vi "TCPtaskhandle.vi"(6 "心跳包":refnum<vi>, 9 "配置信息":refnum<vi>, 10 "状态信息":refnum<vi>, 11 "通信状态":refnum<vi>) -> ()   [LabVIEW 2016, in "数据传输系统.lvlib"]
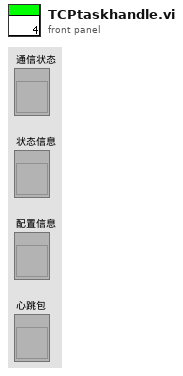
[diagram p1: front panel]
types:
  T1 = cluster{"setini":string, "sysini":string, "hechaini":string, "actualwrite":string, "actualread":string, "datasent":string, "反控命令信息队列":string, "反控与仪器交互":string}
  T2 = cluster{"站点":string, "设备":string, "IP":string, "PORT":string, "MN":string, "PW":string}
  T3 = cluster{"1st Error to Convert ":i32, "步骤 ":enum16{"打开连接", "发送数据", "读取数据", "数据处理", "关闭连接"}, "元素":string, "TCP服务端掉线计数":i32, "TCP掉线时间节点":string}
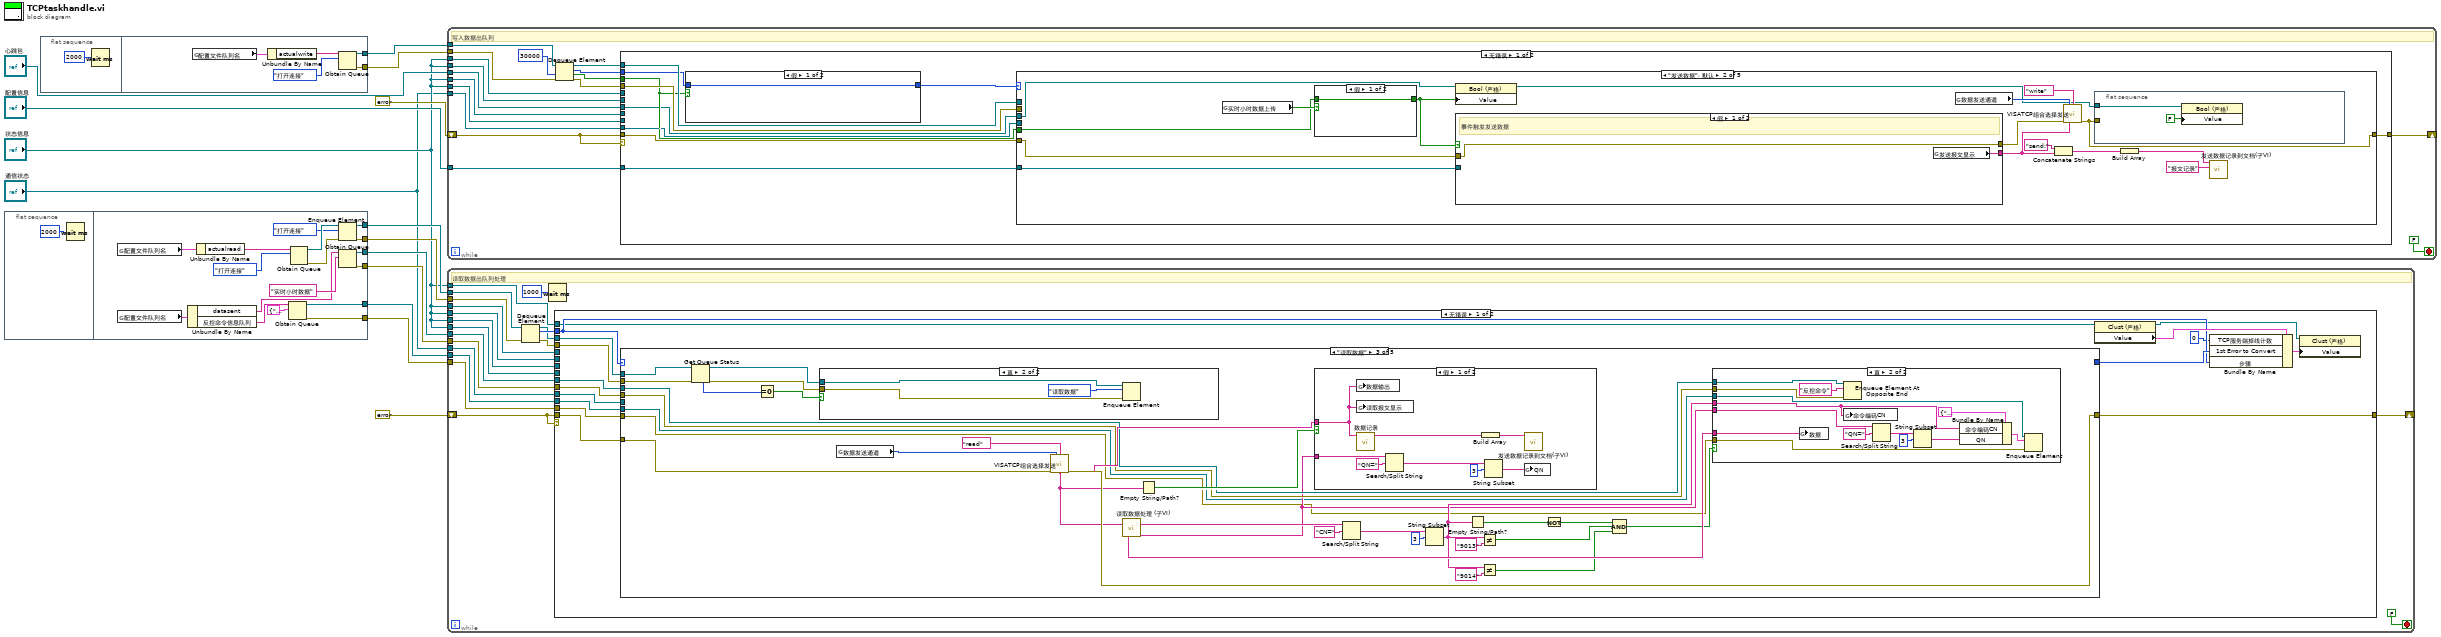
[diagram p0: block diagram]
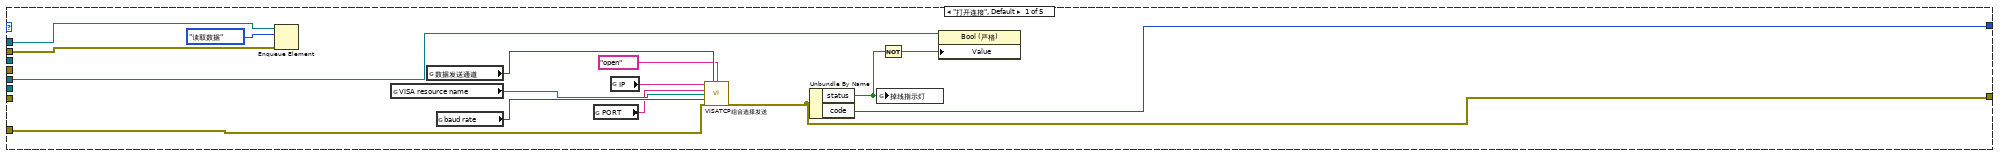
[diagram p2: hidden frame]
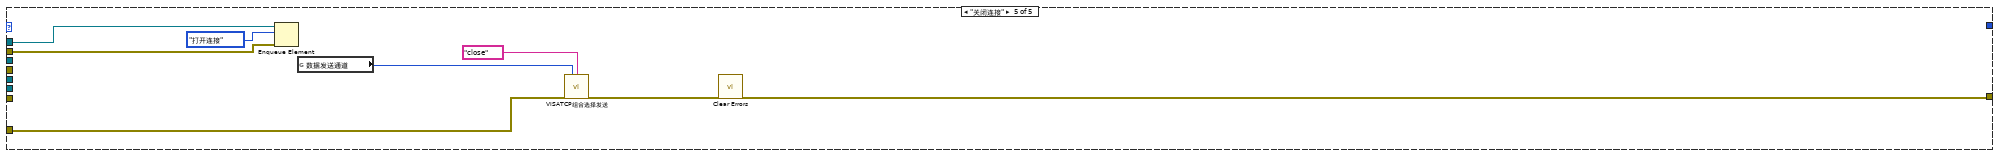
[diagram p8: hidden frame]
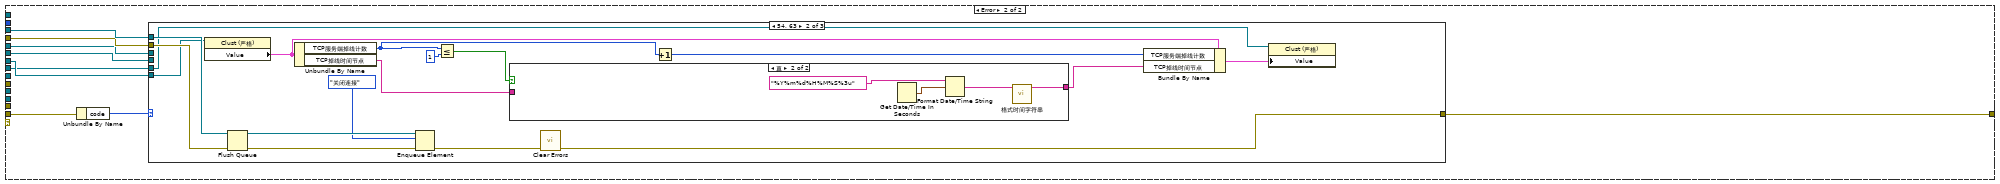
[diagram p9: hidden frame]
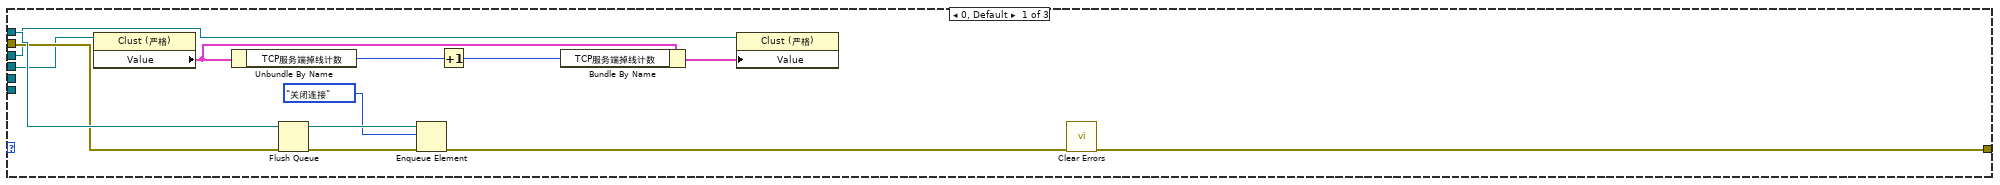
[diagram p10: hidden frame]
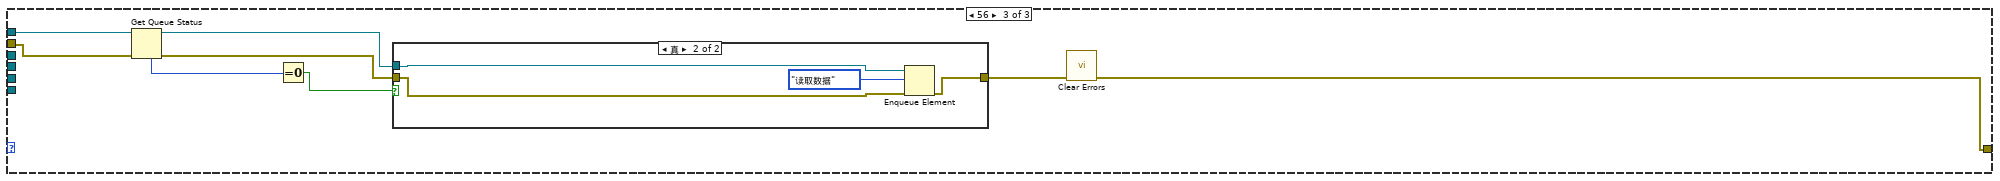
[diagram p12: hidden frame]
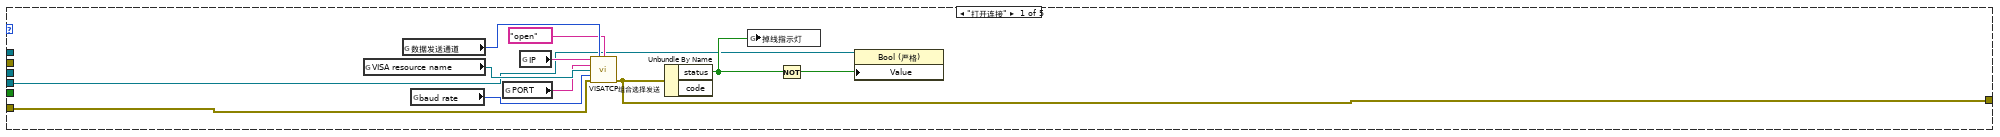
[diagram p14: hidden frame]
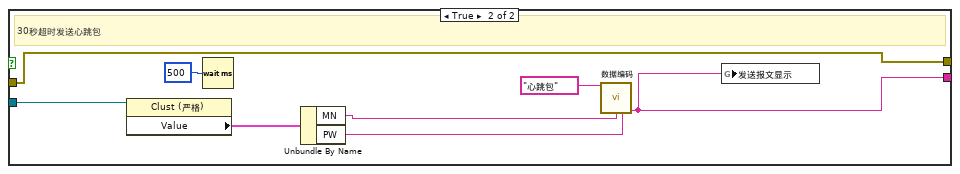
[diagram p15: hidden frame]
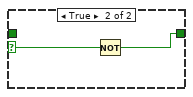
[diagram p16: hidden frame]
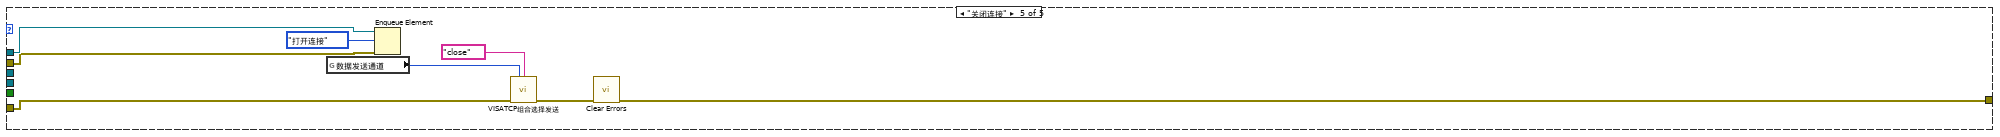
[diagram p19: hidden frame]
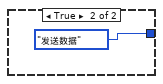
[diagram p20: hidden frame]
diagram:
  n1 = flat-sequence {
    tunnel: [w29] -> w8
    tunnel: [w28] -> w9
    tunnel: [w26] -> w11
    tunnel: [w25] -> w12
    tunnel: [w23] -> w13
    tunnel: [w22] -> w14
    frame #0 {
      n2 = Wait (ms)(milliseconds to wait=u32 2000 ("等待时间（毫秒）")) -> ()  [unwired: 1 out]
    }
    frame #1 {
      n3 = global read "断电保存全局.vi" "配置文件队列名"() -> (w20:T1)
      n4 = global read "断电保存全局.vi" "配置文件队列名"() -> (w18:T1)
      n5 = Unbundle By Name(w18) -> ("datasent"=w17:string, "反控命令信息队列"=w16:string)
      n6 = Unbundle By Name(w20) -> ("actualread"=w19:string)
      n7 = Obtain Queue(name (unnamed)=w16, element data type=cluster{"命令编码CN":string, "QN":string} {"命令编码CN"="", "QN"=""}) -> (queue out=w23:refnum<queue>, error out=w22:errorcluster)  [unwired: 3 in, 1 out]
      n8 = Obtain Queue(name (unnamed)=w19, element data type=enum16{"打开连接", "发送数据", "读取数据", "数据处理", "关闭连接"}."打开连接" ("枚举")) -> (queue out=w32:refnum<queue>, error out=w27:errorcluster)  [unwired: 3 in, 1 out]
      n9 = Enqueue Element(queue=w32, element=enum16{"打开连接", "发送数据", "读取数据", "数据处理", "关闭连接"}."打开连接" ("枚举"), error in (no error)=w27) -> (queue out=w29:refnum<queue>, error out=w28:errorcluster)  [unwired: 1 in, 1 out]
      n10 = Obtain Queue(name (unnamed)=w17, element data type="实时小时数据" ("元素")) -> (queue out=w26:refnum<queue>, error out=w25:errorcluster)  [unwired: 3 in, 1 out]
    }
  }
  n11 = flat-sequence {
    tunnel: [w37] -> w5
    tunnel: [w36] -> w6
    frame #0 {
      n12 = Wait (ms)(milliseconds to wait=u32 2000 ("等待时间（毫秒）")) -> ()  [unwired: 1 out]
    }
    frame #1 {
      n13 = global read "断电保存全局.vi" "配置文件队列名"() -> (w35:T1)
      n14 = Unbundle By Name(w35) -> ("actualwrite"=w34:string)
      n15 = Obtain Queue(name (unnamed)=w34, element data type=enum16{"打开连接", "发送数据", "读取数据", "数据处理", "关闭连接"}."打开连接" ("枚举")) -> (queue out=w37:refnum<queue>, error out=w36:errorcluster)  [unwired: 3 in, 1 out]
    }
  }
  n16 = while {
    tunnel: w5 -> [w54]
    tunnel: w6 -> [w53]
    shift-right: [w49] -> _
    shift-left: errorcluster {"status"=FALSE, "code"=0, "source"=""} ("error out") -> [w48]
    tunnel: "通信状态" -> [w45]
    tunnel: "配置信息" -> [w44]
    tunnel: "心跳包" -> [w43]
    tunnel: "状态信息" -> [w42]
    tunnel: "状态信息" -> [w41]
    tunnel: "状态信息" -> [w40]
    tunnel: "状态信息" -> [w39]
    stop <- FALSE stop-if-true
    # "写入数据出队列"
    n17 = Dequeue Element(queue=w54, timeout in ms (-1)=30000 ("超时毫秒(-1)"), error in (no error)=w53) -> (queue out=w47:refnum<queue>, element=w51:enum16{"打开连接", "发送数据", "读取数据", "数据处理", "关闭连接"}, timed out?=w50:bool, error out=w46:errorcluster)
    n18 = case shown="无错误" w48 {
      tunnel: w51 -> [w59 _]
      tunnel: w50 -> [w61 _]
      tunnel: [w65 w122] -> w49
      tunnel: w48 -> [w64 w126]
      tunnel: w47 -> [w63 w124]
      tunnel: w46 -> [w62 w123]
      tunnel: w45 -> [w58 _]
      tunnel: w44 -> [w57 _]
      tunnel: w43 -> [w56 _]
      tunnel: w42 -> [_ w121]
      tunnel: w41 -> [_ w120]
      tunnel: w40 -> [_ w119]
      tunnel: w39 -> [_ w118]
      frame No Error {
        n19 = case shown="假" w61 {
          tunnel: [w116 enum16{"打开连接", "发送数据", "读取数据", "数据处理", "关闭连接"}."发送数据" ("枚举")] -> w60
          tunnel: w59 -> [w116 _]
          frame False {
          }
          frame True {
          }
        }
        n20 = case shown="\"发送数据\", 默认" w60 {
          tunnel: w61 -> [_ w81 _ _ _]
          tunnel: [w68 w84 _ _ w109] -> w65
          tunnel: w64 -> [w70 w90 _ _ w110]
          tunnel: w63 -> [_ _ _ _ w111]
          tunnel: w62 -> [_ _ _ _ w108]
          tunnel: w58 -> [w66 _ _ _ _]
          tunnel: w57 -> [_ w80 _ _ _]
          tunnel: w56 -> [_ w78 _ _ _]
          frame "打开连接" {
            n21 = global read "断电保存全局.vi" "VISA resource name"() -> (w76:refnum<visa-resource-name>)
            n22 = global read "断电保存全局.vi" "数据发送通道"() -> (w73:enum16{"TCP", "VISA"})
            n23 = global read "断电保存全局.vi" "baud rate"() -> (w75:u32)
            n24 = global read "断电保存全局.vi" "PORT"() -> (w74:string)
            n25 = global read "断电保存全局.vi" "IP"() -> (w72:string)
            n26 = call "VISATCP组合选择发送.vi"("IP"=w72, "数据发送通道"=w73, "命令"="open", "PORT"=w74, "VISA resource name"=w76, "baud rate"=w75, "error in (no error)"=w70) -> ("错误输出"=w68:errorcluster)  [unwired: 5 in, 3 out]
            n27 = Unbundle By Name(w68) -> ("status"=w67:bool)  [unwired: 1 out]
            n28 = global write "全局 数据发送重叠.vi" "掉线指示灯"(w67) -> ()
            n29 = Not(x=w67) -> (.not. x?=w69:bool)
            n30 = property class="Bool (严格)"(reference=w66, "Value"=w69) -> ()  [unwired: 1 in, 2 out]
          }
          frame "发送数据", Default {
            n31 = global read "全局1.vi" "实时小时数据上传"() -> (w82:bool)
            n32 = case shown="假" w82 {
              selector: w82 -> [_ w107]
              tunnel: w81 -> [w105 _]
              tunnel: [w105 w106] -> w79
              frame False {
              }
              frame True {
                n33 = Not(x=w107) -> (.not. x?=w106:bool)
              }
            }
            n34 = property class="Bool (严格)"(reference=w78, "Value"=w79) -> (reference out=w77:refnum<vi>)  [unwired: 1 in, 1 out]
            n35 = case shown="假" w79 {
              tunnel: [w96 w99] -> w86
              tunnel: w90 -> [w95 w100]
              tunnel: [w95 w100] -> w89
              tunnel: w80 -> [_ w97]
              frame False {
                # "事件触发发送数据"
                n36 = global read "全局1.vi" "发送报文显示"() -> (w96:string)
              }
              frame True {
                # "30秒超时发送心跳包"
                n37 = property class="Clust (严格)"(reference=w97) -> ("Value"=w103:T2)  [unwired: 1 in, 2 out]
                n38 = Wait (ms)(milliseconds to wait=u32 500 ("等待时间（毫秒）")) -> ()  [unwired: 1 out]
                n39 = Unbundle By Name(w103) -> ("MN"=w102:string, "PW"=w101:string)
                n40 = call "数据编码.vi"("table输入"="心跳包", "MN"=w102, "PW"=w101) -> ("通讯包字符串"=w99:string)  [unwired: 11 in, 1 out]
                n41 = global write "全局1.vi" "发送报文显示"(w99) -> ()
              }
            }
            n42 = global read "断电保存全局.vi" "数据发送通道"() -> (w91:enum16{"TCP", "VISA"})
            n43 = Concatenate Strings("send:" ("字符串"), w86) -> (w85:string)
            n44 = call "VISATCP组合选择发送.vi"("数据发送通道"=w91, "命令"="write", "error in (no error)"=w89, "写入缓冲区"=w86) -> ("错误输出"=w84:errorcluster)  [unwired: 8 in, 3 out]
            n45 = flat-sequence {
              tunnel: w84 -> [_]
              tunnel: w77 -> [w93]
              frame #0 {
                n46 = property class="Bool (严格)"(reference=w93, "Value"=FALSE ("心跳包")) -> ()  [unwired: 1 in, 2 out]
              }
            }
            n47 = Build Array(w85) -> (w88:string[])
            n48 = call "发送数据记录到文档(子VI).vi"("字符串"="报文记录", "数组"=w88) -> ()  [unwired: 8 in, 1 out]
          }
          frame "读取数据" {
          }
          frame "数据处理" {
          }
          frame "关闭连接" {
            n49 = global read "断电保存全局.vi" "数据发送通道"() -> (w113:enum16{"TCP", "VISA"})
            n50 = Enqueue Element(queue=w111, element=enum16{"打开连接", "发送数据", "读取数据", "数据处理", "关闭连接"}."打开连接" ("枚举"), error in (no error)=w108) -> ()  [unwired: 1 in, 3 out]
            n51 = call "VISATCP组合选择发送.vi"("数据发送通道"=w113, "命令"="close", "error in (no error)"=w110) -> ("错误输出"=w114:errorcluster)  [unwired: 9 in, 3 out]
            n52 = call <vilib>:"Clear Errors.vi"("error in (no error)"=w114) -> ("error out"=w109:errorcluster)  [unwired: 5 in, 1 out]
          }
        }
      }
      frame Error {
        n53 = Unbundle By Name(w126) -> ("code"=w125:i32)
        n54 = case shown="54, 63" w125 {
          tunnel: w124 -> [w135 w153 w165]
          tunnel: w123 -> [w134 w152 w164]
          tunnel: [w133 w150 w163] -> w122
          tunnel: w121 -> [w128 _ _]
          tunnel: w120 -> [w127 _ _]
          tunnel: w119 -> [_ w141 _]
          tunnel: w118 -> [_ w140 _]
          frame 0, Default {
            n55 = property class="Clust (严格)"(reference=w128) -> ("Value"=w132:T3)  [unwired: 1 in, 2 out]
            n56 = Unbundle By Name(w132) -> ("TCP服务端掉线计数"=w130:i32)
            n57 = Flush Queue(queue=w135, error in (no error)=w134) -> (queue out=w137:refnum<queue>, error out=w138:errorcluster)  [unwired: 1 out]
            n58 = Enqueue Element(queue=w137, element=enum16{"打开连接", "发送数据", "读取数据", "数据处理", "关闭连接"}."关闭连接" ("枚举"), error in (no error)=w138) -> (error out=w139:errorcluster)  [unwired: 1 in, 2 out]
            n59 = Increment(x=w130) -> (x+1=w131:i32)
            n60 = Bundle By Name(cluster=w132, "TCP服务端掉线计数"=w131) -> (w129:T3)
            n61 = property class="Clust (严格)"(reference=w127, "Value"=w129) -> ()  [unwired: 1 in, 2 out]
            n62 = call <vilib>:"Clear Errors.vi"("error in (no error)"=w139) -> ("error out"=w133:errorcluster)  [unwired: 5 in, 1 out]
          }
          frame 54, 63 {
            n63 = property class="Clust (严格)"(reference=w141) -> ("Value"=w145:T3)  [unwired: 1 in, 2 out]
            n64 = Flush Queue(queue=w153, error in (no error)=w152) -> (queue out=w155:refnum<queue>, error out=w156:errorcluster)  [unwired: 1 out]
            n65 = Unbundle By Name(w145) -> ("TCP服务端掉线计数"=w149:i32, "TCP掉线时间节点"=w142:string)
            n66 = Enqueue Element(queue=w155, element=enum16{"打开连接", "发送数据", "读取数据", "数据处理", "关闭连接"}."关闭连接" ("枚举"), error in (no error)=w156) -> (error out=w151:errorcluster)  [unwired: 1 in, 2 out]
            n67 = Less Or Equal?(x=w149, y=1) -> (x <= y?=w147:bool)
            n68 = case shown="真" w147 {
              tunnel: [w157 w158] -> w146
              tunnel: w142 -> [w157 _]
              frame False {
              }
              frame True {
                n69 = Get Date/Time In Seconds() -> (seconds since 1Jan1904=w159:timestamp)
                n70 = Format Date/Time String(time format string (%c)="%Y%m%d%H%M%S%3u" ("时间格式字符串(%c)"), seconds (now)=w159) -> (date/time string=w161:string)  [unwired: 1 in]
                n71 = call "格式时间字符串.vi"("字符串"=w161) -> ("连接的字符串"=w158:string)  [unwired: 10 in]
              }
            }
            n72 = call <vilib>:"Clear Errors.vi"("error in (no error)"=w151) -> ("error out"=w150:errorcluster)  [unwired: 5 in, 1 out]
            n73 = Increment(x=w149) -> (x+1=w144:i32)
            n74 = Bundle By Name(cluster=w145, "TCP服务端掉线计数"=w144, "TCP掉线时间节点"=w146) -> (w143:T3)
            n75 = property class="Clust (严格)"(reference=w140, "Value"=w143) -> ()  [unwired: 1 in, 2 out]
          }
          frame 56 {
            n76 = Flush Queue(queue=w165, error in (no error)=w164) -> (error out=w162:errorcluster)  [unwired: 2 out]
            n77 = call <vilib>:"Clear Errors.vi"("error in (no error)"=w162) -> ("error out"=w163:errorcluster)  [unwired: 5 in, 1 out]
          }
        }
      }
    }
  }
  n78 = while {
    tunnel: w8 -> [w184]
    tunnel: w9 -> [w183]
    shift-right: [w180] -> _
    shift-left: errorcluster {"status"=FALSE, "code"=0, "source"=""} ("error out") -> [w179]
    tunnel: w11 -> [w175]
    tunnel: w12 -> [w174]
    tunnel: w13 -> [w173]
    tunnel: w14 -> [w172]
    tunnel: "状态信息" -> [w171]
    tunnel: "状态信息" -> [w170]
    tunnel: "状态信息" -> [w169]
    tunnel: "状态信息" -> [w168]
    tunnel: "状态信息" -> [w167]
    tunnel: "通信状态" -> [w166]
    stop <- FALSE stop-if-true
    # "读取数据出队列处理"
    n79 = Dequeue Element(queue=w184, error in (no error)=w183) -> (queue out=w178:refnum<queue>, element=w181:enum16{"打开连接", "发送数据", "读取数据", "数据处理", "关闭连接"}, error out=w177:errorcluster)  [unwired: 1 in, 1 out]
    n80 = Wait (ms)(milliseconds to wait=u32 1000 ("等待时间（毫秒）")) -> ()  [unwired: 1 out]
    n81 = case shown="无错误" w179 {
      tunnel: w181 -> [w194 _]
      tunnel: [w200 w283] -> w180
      tunnel: w179 -> [w199 w287]
      tunnel: w178 -> [w198 w285]
      tunnel: w177 -> [w197 w284]
      tunnel: w175 -> [w192 _]
      tunnel: w174 -> [w191 _]
      tunnel: w173 -> [w190 _]
      tunnel: w172 -> [w189 _]
      tunnel: w171 -> [w188 _]
      tunnel: w170 -> [_ w282]
      tunnel: w169 -> [_ w281]
      tunnel: w168 -> [_ w280]
      tunnel: w167 -> [_ w279]
      tunnel: w166 -> [w185 _]
      frame No Error {
        n82 = case shown="\"读取数据\"" w194 {
          tunnel: [w209 _ w242 _ w274] -> w200
          tunnel: w199 -> [w208 _ w245 _ w275]
          tunnel: w198 -> [w206 _ w237 _ w272]
          tunnel: w197 -> [w205 _ w236 _ w271]
          tunnel: [w204 _ _ _ _] -> w195
          tunnel: w192 -> [_ _ w229 _ _]
          tunnel: w191 -> [_ _ w228 _ _]
          tunnel: w190 -> [_ _ w217 _ _]
          tunnel: w189 -> [_ _ w216 _ _]
          tunnel: w185 -> [w202 _ _ _ _]
          frame "打开连接", Default {
            n83 = Enqueue Element(queue=w206, element=enum16{"打开连接", "发送数据", "读取数据", "数据处理", "关闭连接"}."读取数据" ("枚举"), error in (no error)=w205) -> ()  [unwired: 1 in, 3 out]
            n84 = global read "断电保存全局.vi" "VISA resource name"() -> (w215:refnum<visa-resource-name>)
            n85 = global read "断电保存全局.vi" "数据发送通道"() -> (w212:enum16{"TCP", "VISA"})
            n86 = global read "断电保存全局.vi" "baud rate"() -> (w214:u32)
            n87 = global read "断电保存全局.vi" "PORT"() -> (w213:string)
            n88 = global read "断电保存全局.vi" "IP"() -> (w211:string)
            n89 = call "VISATCP组合选择发送.vi"("IP"=w211, "数据发送通道"=w212, "命令"="open", "PORT"=w213, "VISA resource name"=w215, "baud rate"=w214, "error in (no error)"=w208) -> ("错误输出"=w209:errorcluster)  [unwired: 5 in, 3 out]
            n90 = Unbundle By Name(w209) -> ("status"=w203:bool, "code"=w204:i32)
            n91 = global write "全局 数据发送重叠.vi" "掉线指示灯"(w203) -> ()
            n92 = Not(x=w203) -> (.not. x?=w201:bool)
            n93 = property class="Bool (严格)"(reference=w202, "Value"=w201) -> ()  [unwired: 1 in, 2 out]
          }
          frame "发送数据" {
          }
          frame "读取数据" {
            n94 = Get Queue Status(queue=w237, error in (no error)=w236) -> (queue out=w233:refnum<queue>, error out=w232:errorcluster, # elements in queue=w235:i32)  [unwired: 1 in, 5 out]
            n95 = Equal To 0?(x=w235) -> (x = 0?=w234:bool)
            n96 = case shown="真" w234 {
              tunnel: w233 -> [_ w269]
              tunnel: w232 -> [_ w268]
              frame False {
              }
              frame True {
                n97 = Enqueue Element(queue=w269, element=enum16{"打开连接", "发送数据", "读取数据", "数据处理", "关闭连接"}."读取数据" ("枚举"), error in (no error)=w268) -> ()  [unwired: 1 in, 3 out]
              }
            }
            n98 = global read "断电保存全局.vi" "数据发送通道"() -> (w244:enum16{"TCP", "VISA"})
            n99 = call "VISATCP组合选择发送.vi"("数据发送通道"=w244, "命令"="read", "error in (no error)"=w245) -> ("读取缓冲区"=w230:string, "错误输出"=w242:errorcluster)  [unwired: 9 in, 2 out]
            n100 = call "读取数据处理 (子VI).vi"("data out"=w230) -> ("命令编码CN"=w238:string, "数据"=w226:string, "时间QN"=w218:string)  [unwired: 8 in, 4 out]
            n101 = Empty String/Path?(string/path=w230) -> (empty?=w231:bool)
            n102 = case shown="假" w231 {
              tunnel: w230 -> [w265 _]
              tunnel: w218 -> [w262 _]
              frame False {
                n103 = global write "全局1.vi" "数据输出"(w265) -> ()
                n104 = global write "全局1.vi" "读取报文显示"(w265) -> ()
                n105 = call "数据记录.vi"("写入字段"=w265) -> ("连接的字符串"=w266:string)  [unwired: 10 in]
                n106 = Search/Split String(string=w262, search string/char (-)="QN=" ("搜索字符串/字符(-)")) -> (match + rest of string=w261:string)  [unwired: 1 in, 2 out]
                n107 = Build Array(w266) -> (w267:string[])
                n108 = String Subset(string=w261, offset (0)=3 ("偏移量(0)")) -> (substring=w260:string)  [unwired: 1 in]
                n109 = call "发送数据记录到文档(子VI).vi"("数组"=w267) -> ()  [unwired: 9 in, 1 out]
                n110 = global write "全局1.vi" "QN"(w260) -> ()
              }
              frame True {
              }
            }
            n111 = Search/Split String(string=w238, search string/char (-)="CN=" ("搜索字符串/字符(-)")) -> (match + rest of string=w239:string)  [unwired: 1 in, 2 out]
            n112 = String Subset(string=w239, offset (0)=3 ("偏移量(0)")) -> (substring=w224:string)  [unwired: 1 in]
            n113 = Empty String/Path?(string/path=w224) -> (empty?=w227:bool)
            n114 = Not Equal?(x=w224, y="9013") -> (x != y?=w221:bool)
            n115 = Not Equal?(x=w224, y="9014") -> (x != y?=w220:bool)
            n116 = Not(x=w227) -> (.not. x?=w219:bool)
            n117 = Compound Arithmetic op=AND ("复合运算")(w219, w221, w220) -> (w225:bool)
            n118 = case shown="真" w225 {
              tunnel: w229 -> [_ w259]
              tunnel: w228 -> [_ w258]
              tunnel: w226 -> [_ w257]
              tunnel: w224 -> [_ w248]
              tunnel: w218 -> [_ w253]
              tunnel: w217 -> [_ w252]
              tunnel: w216 -> [_ w251]
              frame False {
              }
              frame True {
                n119 = global write "全局1.vi" "数据"(w257) -> ()
                n120 = Enqueue Element At Opposite End(queue=w259, element="反控命令" ("元素"), error in (no error)=w258) -> ()  [unwired: 1 in, 3 out]
                n121 = global write "全局1.vi" "命令编码CN"(w248) -> ()
                n122 = Search/Split String(string=w253, search string/char (-)="QN=" ("搜索字符串/字符(-)")) -> (match + rest of string=w256:string)  [unwired: 1 in, 2 out]
                n123 = String Subset(string=w256, offset (0)=3 ("偏移量(0)")) -> (substring=w247:string)  [unwired: 1 in]
                n124 = Bundle By Name(cluster=cluster{"命令编码CN":string, "QN":string} {"命令编码CN"="", "QN"=""}, "命令编码CN"=w248, "QN"=w247) -> (w249:cluster{"命令编码CN":string, "QN":string})
                n125 = Enqueue Element(queue=w252, element=w249, error in (no error)=w251) -> ()  [unwired: 1 in, 3 out]
              }
            }
          }
          frame "数据处理" {
          }
          frame "关闭连接" {
            n126 = Enqueue Element(queue=w272, element=enum16{"打开连接", "发送数据", "读取数据", "数据处理", "关闭连接"}."打开连接" ("枚举"), error in (no error)=w271) -> ()  [unwired: 1 in, 3 out]
            n127 = global read "断电保存全局.vi" "数据发送通道"() -> (w277:enum16{"TCP", "VISA"})
            n128 = call "VISATCP组合选择发送.vi"("数据发送通道"=w277, "命令"="close", "error in (no error)"=w275) -> ("错误输出"=w276:errorcluster)  [unwired: 9 in, 3 out]
            n129 = call <vilib>:"Clear Errors.vi"("error in (no error)"=w276) -> ("error out"=w274:errorcluster)  [unwired: 5 in, 1 out]
          }
        }
        n130 = property class="Clust (严格)"(reference=w188) -> (reference out=w187:refnum<vi>, "Value"=w196:T3)  [unwired: 1 in, 1 out]
        n131 = Bundle By Name(cluster=w196, "TCP服务端掉线计数"=0, "1st Error to Convert"=w195, "步骤"=w194) -> (w186:T3)
        n132 = property class="Clust (严格)"(reference=w187, "Value"=w186) -> ()  [unwired: 1 in, 2 out]
      }
      frame Error {
        n133 = Unbundle By Name(w287) -> ("code"=w286:i32)
        n134 = case shown="54, 63" w286 {
          tunnel: w285 -> [w296 w314 w324]
          tunnel: w284 -> [w295 w313 w323]
          tunnel: [w294 w311 w330] -> w283
          tunnel: w282 -> [w289 _ _]
          tunnel: w281 -> [w288 _ _]
          tunnel: w280 -> [_ w302 _]
          tunnel: w279 -> [_ w301 _]
          frame 0, Default {
            n135 = property class="Clust (严格)"(reference=w289) -> ("Value"=w293:T3)  [unwired: 1 in, 2 out]
            n136 = Unbundle By Name(w293) -> ("TCP服务端掉线计数"=w291:i32)
            n137 = Flush Queue(queue=w296, error in (no error)=w295) -> (queue out=w298:refnum<queue>, error out=w299:errorcluster)  [unwired: 1 out]
            n138 = Enqueue Element(queue=w298, element=enum16{"打开连接", "发送数据", "读取数据", "数据处理", "关闭连接"}."关闭连接" ("枚举"), error in (no error)=w299) -> (error out=w300:errorcluster)  [unwired: 1 in, 2 out]
            n139 = Increment(x=w291) -> (x+1=w292:i32)
            n140 = Bundle By Name(cluster=w293, "TCP服务端掉线计数"=w292) -> (w290:T3)
            n141 = property class="Clust (严格)"(reference=w288, "Value"=w290) -> ()  [unwired: 1 in, 2 out]
            n142 = call <vilib>:"Clear Errors.vi"("error in (no error)"=w300) -> ("error out"=w294:errorcluster)  [unwired: 5 in, 1 out]
          }
          frame 54, 63 {
            n143 = property class="Clust (严格)"(reference=w302) -> ("Value"=w306:T3)  [unwired: 1 in, 2 out]
            n144 = Flush Queue(queue=w314, error in (no error)=w313) -> (queue out=w316:refnum<queue>, error out=w317:errorcluster)  [unwired: 1 out]
            n145 = Unbundle By Name(w306) -> ("TCP服务端掉线计数"=w310:i32, "TCP掉线时间节点"=w303:string)
            n146 = Enqueue Element(queue=w316, element=enum16{"打开连接", "发送数据", "读取数据", "数据处理", "关闭连接"}."关闭连接" ("枚举"), error in (no error)=w317) -> (error out=w312:errorcluster)  [unwired: 1 in, 2 out]
            n147 = Less Or Equal?(x=w310, y=1) -> (x <= y?=w308:bool)
            n148 = case shown="真" w308 {
              tunnel: [w318 w319] -> w307
              tunnel: w303 -> [w318 _]
              frame False {
              }
              frame True {
                n149 = Get Date/Time In Seconds() -> (seconds since 1Jan1904=w320:timestamp)
                n150 = Format Date/Time String(time format string (%c)="%Y%m%d%H%M%S%3u" ("时间格式字符串(%c)"), seconds (now)=w320) -> (date/time string=w322:string)  [unwired: 1 in]
                n151 = call "格式时间字符串.vi"("字符串"=w322) -> ("连接的字符串"=w319:string)  [unwired: 10 in]
              }
            }
            n152 = call <vilib>:"Clear Errors.vi"("error in (no error)"=w312) -> ("error out"=w311:errorcluster)  [unwired: 5 in, 1 out]
            n153 = Increment(x=w310) -> (x+1=w305:i32)
            n154 = Bundle By Name(cluster=w306, "TCP服务端掉线计数"=w305, "TCP掉线时间节点"=w307) -> (w304:T3)
            n155 = property class="Clust (严格)"(reference=w301, "Value"=w304) -> ()  [unwired: 1 in, 2 out]
          }
          frame 56 {
            n156 = Get Queue Status(queue=w324, error in (no error)=w323) -> (queue out=w326:refnum<queue>, error out=w325:errorcluster, # elements in queue=w328:i32)  [unwired: 1 in, 5 out]
            n157 = Equal To 0?(x=w328) -> (x = 0?=w327:bool)
            n158 = case shown="真" w327 {
              tunnel: [w331 w334] -> w329
              tunnel: w326 -> [_ w333]
              tunnel: w325 -> [w331 w332]
              frame False {
              }
              frame True {
                n159 = Enqueue Element(queue=w333, element=enum16{"打开连接", "发送数据", "读取数据", "数据处理", "关闭连接"}."读取数据" ("枚举"), error in (no error)=w332) -> (error out=w334:errorcluster)  [unwired: 1 in, 2 out]
              }
            }
            n160 = call <vilib>:"Clear Errors.vi"("error in (no error)"=w329) -> ("error out"=w330:errorcluster)  [unwired: 5 in, 1 out]
          }
        }
      }
    }
  }
